vi "Parse Conditional Disable Symbols.vi"(8 "Target Name":string, 11 "CCSymbols Value":variant) -> (1 "Values":string[](array[string]), 2 "Symbols":string[](array[string]), 3 "Targets":string[](array[string]))   [LabVIEW 2023, in "VIDoc Parsing.lvlib" / "Project Documentation.lvclass"]
uses:
  Project Documentation.lvclass
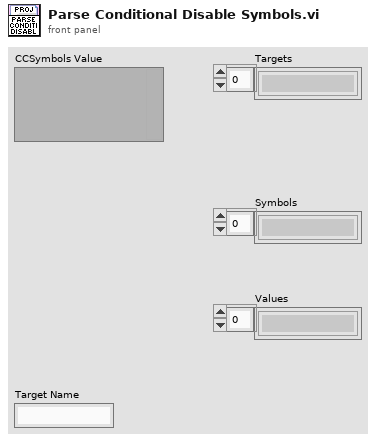
[diagram p1: front panel]
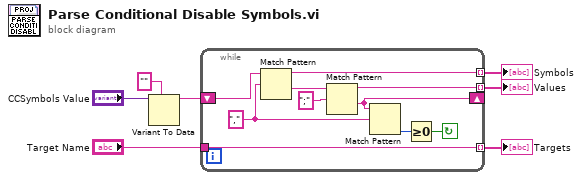
[diagram p0: block diagram]
diagram:
  n1 = Variant To Data(type="", Variant="CCSymbols Value") -> (data=w4:string)  [unwired: 1 in, 1 out]
  n2 = while {
    shift-right: [w12] -> _
    shift-left: w4 -> [w17]
    tunnel: [w14] -> w7 mode=indexing
    tunnel: [w13] -> w2 mode=indexing
    tunnel: "Target Name" -> [w8]
    tunnel: [w8] -> w1 mode=indexing
    stop <- w9 continue-if-true
    w11 = "," ("regular expression")
    n3 = Match Pattern(string=w17, regular expression=w11) -> (before substring=w14:string, after substring=w16:string)  [unwired: 1 in, 2 out]
    n4 = Match Pattern(string=w16, regular expression=";") -> (before substring=w13:string, after substring=w12:string)  [unwired: 1 in, 2 out]
    n5 = Match Pattern(string=w12, regular expression=w11) -> (offset past match=w10:i32)  [unwired: 1 in, 3 out]
    n6 = Greater Or Equal To 0?(x=w10) -> (x >= 0?=w9:bool)
  }
  "Symbols" <- w7
  "Values" <- w2
  "Targets" <- w1
